vi "Theta Drive_Two step on.vi"(8 "error in (no error)":errorcluster, 9 "Start Location Step (-90to90)":i32, 10 "Target Step (-90to90)":i32, 11 "stop":bool) -> (0 "error out":errorcluster, 1 "Current Motor Step (0to3)":i32, 2 "Current Step (-90to90)":i32, 3 "Boolean array":bool[](array[boolean]))   [LabVIEW 2017]
uses:
  <vilib>/myRIO/Instrument Drivers/Onboard IO/DIO/typedefs/DIO Reference.ctl
  <vilib>/myRIO/Common/Instrument Driver Framework/Utilities/typedefs/myRIO Generic Hardware Reference.ctl
  <vilib>/myRIO/Common/Instrument Driver Framework/Utilities/typedefs/Hardware Version Enum.ctl
  <vilib>/myRIO/Common/Instrument Driver Framework/Utilities/typedefs/myRIO v1.0 Reference.ctl
  <vilib>/myRIO/Common/Instrument Driver Framework/Utilities/typedefs/Generic FPGA Reference.ctl
  <vilib>/myRIO/Common/Instrument Driver Framework/myRIO v1.0/DIO/typedefs/DIO Channels List.ctl
  <vilib>/myRIO/Common/Instrument Driver Framework/myRIO v1.0/DIO/typedefs/DIO Channels Enum.ctl
  <vilib>/userdefined/High Color/nirio_resource_hc.ctl
  <vilib>/myRIO/Common/Instrument Driver Framework/Utilities/vis/Is FPGA Ref Available.vi
  <vilib>/myRIO/Common/Instrument Driver Framework/myRIO v1.0/DIO/vis/myRIO v1.1 Open DIO.vi
  <vilib>/myRIO/Instrument Drivers/Onboard IO/DIO/vis/Write.vi
  <vilib>/myRIO/Common/Instrument Driver Framework/Utilities/vis/Validate Channels.vi
  <vilib>/myRIO/Common/Instrument Driver Framework/myRIO v1.0/DIO/vis/myRIO v1.0 Reserve DIO.vi
  <vilib>/myRIO/Common/Instrument Driver Framework/myRIO v1.0/Resource Manager/vis/myRIO v1.0 Reserve Channel List.vi
  <vilib>/myRIO/Common/Instrument Driver Framework/myRIO v1.0/DIO/vis/myRIO v1.0 Build MUX Configuration DIO.vi
  <vilib>/myRIO/Common/Instrument Driver Framework/myRIO v1.0/Resource Manager/vis/myRIO v1.0 Reserve Channel.vi
  <vilib>/myRIO/Common/Instrument Driver Framework/myRIO v1.0/Resource Manager/vis/myRIO v1.0 Unreserve Channel.vi
  <vilib>/myRIO/Common/Instrument Driver Framework/myRIO v1.0/Resource Manager/vis/myRIO v1.0 Create Configuration List.vi
  <vilib>/myRIO/Common/Instrument Driver Framework/myRIO v1.0/Resource Manager/vis/myRIO v1.0 Build Mutex Name.vi
  <vilib>/Utility/VariantDataType/GetNumericInfo.vi
  <vilib>/Utility/error.llb/Error Cluster From Error Code.vi
  <vilib>/myRIO/Common/Instrument Driver Framework/myRIO v1.0/myRIO v1.1 Open.vi
  <vilib>/myRIO/Common/Instrument Driver Framework/Utilities/vis/IO Manager.vi
  <vilib>/myRIO/Common/Instrument Driver Framework/Utilities/vis/Configuration Manager.vi
  <vilib>/myRIO/Common/Instrument Driver Framework/myRIO v1.0/Resource Manager/vis/myRIO v1.0 Configure IO.vi
  <vilib>/myRIO/Common/Instrument Driver Framework/myRIO v1.0/myRIO v1.0 Close.vi
  <vilib>/myRIO/Common/Instrument Driver Framework/myRIO v1.0/DIO/vis/myRIO v1.0 Write DIO.vi
  <vilib>/myRIO/Express VI/Onboard IO/DO/DO Express VI.xnode
  <vilib>/myRIO/Instrument Drivers/Onboard IO/DIO/vis/myRIO DIO Open.xnode
  <vilib>/myRIO/Instrument Drivers/Onboard IO/DIO/DIO.lvlib
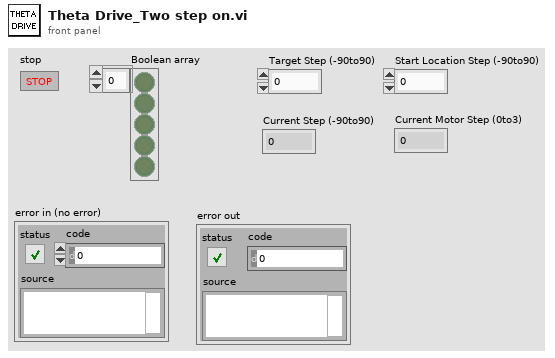
[diagram p1: front panel]
types:
  T1 = typedef "DIO.lvlib/DIO Reference.ctl" = cluster{"myRIO Reference":T2, "DIO Channels List":T6}
  T2 = typedef "myRIO Generic Hardware Reference.ctl" = cluster{"myRIO Model":T3, "myRIO Hardware Reference":T4}
  T3 = typedef "Hardware Version Enum.ctl" = enum16{"Unknown", "myRIO-1900", "myRIO-1950", "roboRIO", "NI ELVIS RIO CM"}
  T4 = typedef "myRIO v1.0 Reference.ctl" = cluster{"Generic FPGA Reference":T5, "Allow multiple opens":bool}
  T5 = typedef "Generic FPGA Reference.ctl" = refnum<k20>
  T6 = typedef "DIO Channels List.ctl" = T7[]
  T7 = typedef "DIO Channels Enum.ctl" = enum16{"Not Connected", "C/DIO0", "C/DIO1", "C/DIO2", "C/DIO3", "C/DIO4", "C/DIO5", "C/DIO6", "C/DIO7", "A/DIO0", "A/DIO1", "A/DIO2", "A/DIO3", "A/DIO4", "A/DIO5", "A/DIO6", "A/DIO7", "A/DIO8", "A/DIO9", "A/DIO10", "A/DIO11", "A/DIO12", "A/DIO13", "A/DIO14", "A/DIO15", "B/DIO0", "B/DIO1", "B/DIO2", "B/DIO3", "B/DIO4", "B/DIO5", "B/DIO6", "B/DIO7", "B/DIO8", "B/DIO9", "B/DIO10", "B/DIO11", "B/DIO12", "B/DIO13", "B/DIO14", "B/DIO15", "LED0", "LED1", "LED2", "LED3", "Button0", "DIO/DIO0", "DIO/DIO1", "DIO/DIO2", "DIO/DIO3", "DIO/DIO4", "DIO/DIO5", "DIO/DIO6", "DIO/DIO7", "DIO/DIO8", "DIO/DIO9", "SPI/CS0", "SPI/CS1", "SPI/CS2", "SPI/CS3", "LED RADIO (Green)", "LED RADIO (Red)", "LED COMM (Green)", "LED COMM (Red)", "LED MODE (Green)", "LED MODE (Red)"}
  T8 = typedef "nirio_resource_hc.ctl" = tag
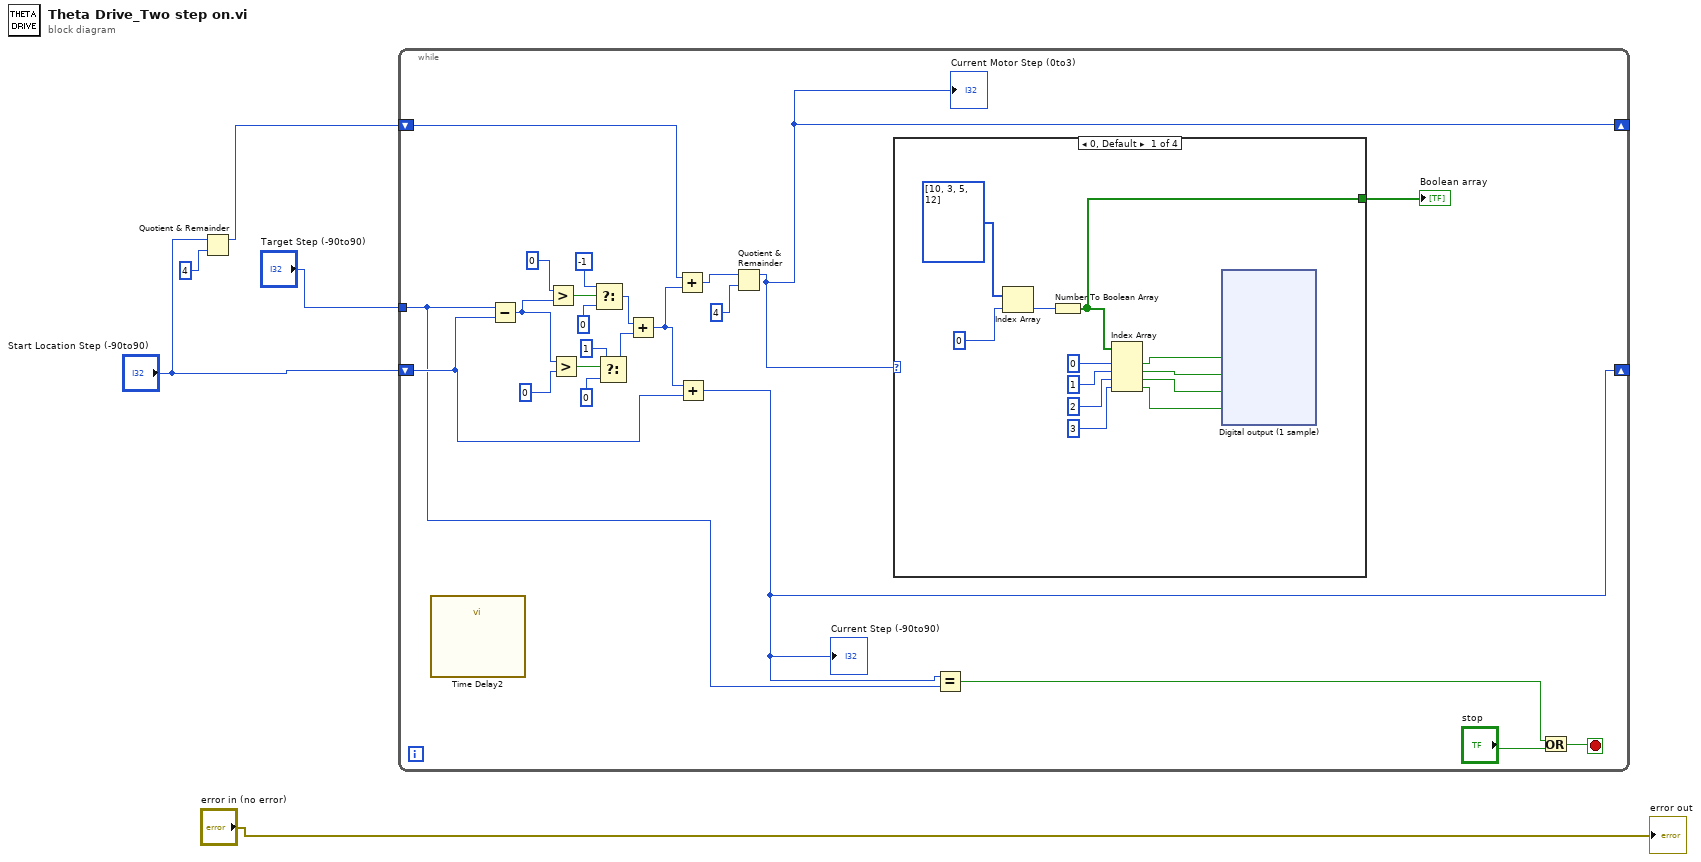
[diagram p0: block diagram]
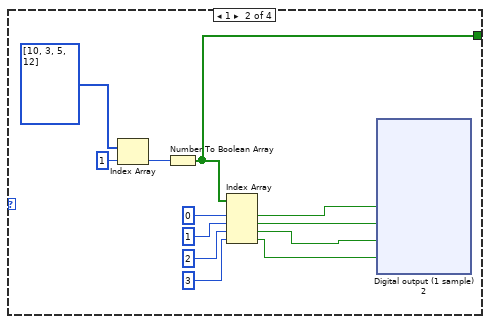
[diagram p2: hidden frame]
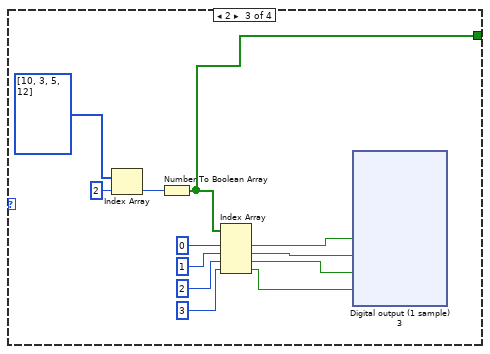
[diagram p3: hidden frame]
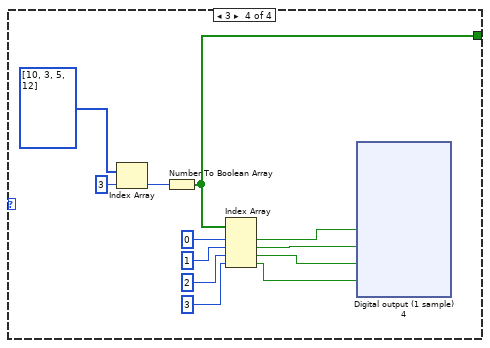
[diagram p4: hidden frame]
diagram:
  n1 = Quotient & Remainder(x="Start Location Step (-90to90)", y=4) -> (x-y*floor(x/y)=w2:i32)  [unwired: 1 out]
  n2 = while {
    shift-right: [w10] -> _
    shift-left: "Start Location Step (-90to90)" -> [w11]
    tunnel: "Target Step (-90to90)" -> [w9]
    shift-right: [w13] -> _
    shift-left: w2 -> [w14]
    stop <- w8 stop-if-true
    n3 = call "Time Delay2"() -> ()  [unwired: 11 in, 1 out]
    n4 = Subtract(x=w9, y=w11) -> (x-y=w26:i32)
    n5 = Greater?(x=0, y=w26) -> (0:w24:bool)
    n6 = Greater?(x=w26, y=0) -> (0:w21:bool)
    n7 = Select(t=-1, s=w24, f=0) -> (s? t:f=w18:i32)
    n8 = Select(t=1, s=w21, f=0) -> (s? t:f=w17:i32)
    n9 = Add(x=w18, y=w17) -> (x+y=w12:i32)
    n10 = Add(x=w14, y=w12) -> (x+y=w16:i32)
    n11 = Add(x=w12, y=w11) -> (x+y=w10:i32)
    "Current Step (-90to90)" <- w10
    n12 = Quotient & Remainder(x=w16, y=4) -> (x-y*floor(x/y)=w13:i32)  [unwired: 1 out]
    "Current Motor Step (0to3)" <- w13
    n13 = case shown="0, Default" w13 {
      tunnel: [w36 w81 w130 w180] -> w28
      frame 0, Default {
        n14 = Index Array(array=i32[] [10, 3, 5, 12], index=0) -> (element=w35:i32)
        n15 = Number To Boolean Array(number=w35) -> (Boolean array=w36:bool[])
        n16 = Index Array(array=w36, index #1=0 ("index"), index #2=1 ("index"), index #3=2 ("index"), index #4=3 ("index")) -> (element #1=w32:bool, element #2=w31:bool, element #3=w30:bool, element #4=w29:bool)
        n17 = xnode "Digital output (1 sample)"("A/DIO0 (Pin 11)"=w32, "A/DIO1 (Pin 13)"=w31, "A/DIO2 (Pin 15)"=w30, "A/DIO3 (Pin 17)"=w29) -> ()  [unwired: 1 in, 1 out]
      }
      frame 1 {
        n18 = Index Array(array=i32[] [10, 3, 5, 12], index=1) -> (element=w82:i32)
        n19 = Number To Boolean Array(number=w82) -> (Boolean array=w81:bool[])
        n20 = Index Array(array=w81, index #1=0 ("index"), index #2=1 ("index"), index #3=2 ("index"), index #4=3 ("index")) -> (element #1=w90:bool, element #2=w89:bool, element #3=w88:bool, element #4=w87:bool)
        n21 = xnode "Digital output (1 sample) 2"("A/DIO0 (Pin 11)"=w90, "A/DIO1 (Pin 13)"=w89, "A/DIO2 (Pin 15)"=w88, "A/DIO3 (Pin 17)"=w87) -> ()  [unwired: 1 in, 1 out]
      }
      frame 2 {
        n22 = Index Array(array=i32[] [10, 3, 5, 12], index=2) -> (element=w132:i32)
        n23 = Number To Boolean Array(number=w132) -> (Boolean array=w130:bool[])
        n24 = Index Array(array=w130, index #1=0 ("index"), index #2=1 ("index"), index #3=2 ("index"), index #4=3 ("index")) -> (element #1=w140:bool, element #2=w139:bool, element #3=w138:bool, element #4=w137:bool)
        n25 = xnode "Digital output (1 sample) 3"("A/DIO0 (Pin 11)"=w140, "A/DIO1 (Pin 13)"=w139, "A/DIO2 (Pin 15)"=w138, "A/DIO3 (Pin 17)"=w137) -> ()  [unwired: 1 in, 1 out]
      }
      frame 3 {
        n26 = Index Array(array=i32[] [10, 3, 5, 12], index=3) -> (element=w182:i32)
        n27 = Number To Boolean Array(number=w182) -> (Boolean array=w180:bool[])
        n28 = Index Array(array=w180, index #1=0 ("index"), index #2=1 ("index"), index #3=2 ("index"), index #4=3 ("index")) -> (element #1=w190:bool, element #2=w189:bool, element #3=w188:bool, element #4=w187:bool)
        n29 = xnode "Digital output (1 sample) 4"("A/DIO0 (Pin 11)"=w190, "A/DIO1 (Pin 13)"=w189, "A/DIO2 (Pin 15)"=w188, "A/DIO3 (Pin 17)"=w187) -> ()  [unwired: 1 in, 1 out]
      }
    }
    "Boolean array" <- w28
    n30 = Equal?(x=w10, y=w9) -> (x = y?=w6:bool)
    n31 = Or(x=w6, y="stop") -> (x .or. y?=w8:bool)
  }
  "error out" <- "error in (no error)"
